vi "Read Waveform data.vi"(8 "error in (no error)":errorcluster, 11 "1D wfm (DBL) Result in":refnum<class "1D wfm (DBL) Result.lvclass">) -> (0 "error out":errorcluster, 2 "Waveform data":waveform(dbl), 3 "1D wfm (DBL) Result out":refnum<class "1D wfm (DBL) Result.lvclass">)   [LabVIEW 2015, in "1D wfm (DBL) Result.lvclass"]
uses:
  1D wfm (DBL) Result.lvclass
  1D wfm (DBL) Result.lvclass/1D wfm (DBL) Result.ctl
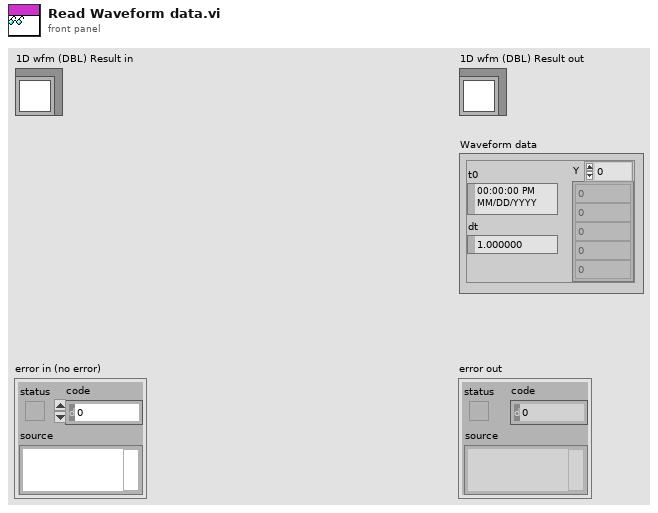
[diagram p1: front panel]
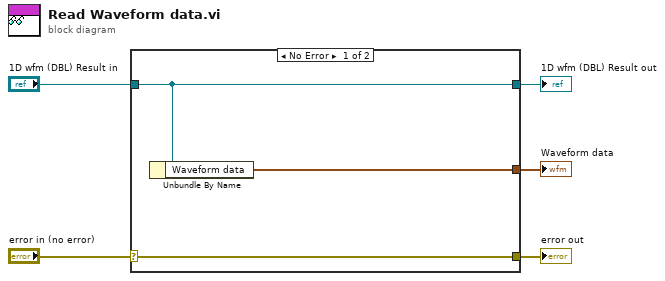
[diagram p0: block diagram]
diagram:
  n1 = case shown="No Error" "error in (no error)" {
    selector: "error in (no error)" -> [w8 w9]
    tunnel: [w8 w9] -> w4
    tunnel: [w7 w10] -> w2
    tunnel: "1D wfm (DBL) Result in" -> [w7 w10]
    tunnel: [w6 _] -> w1
    frame No Error {
      n2 = Unbundle By Name(w7) -> ("Waveform data"=w6:waveform(dbl))
    }
    frame Error {
    }
  }
  "error out" <- w4
  "1D wfm (DBL) Result out" <- w2
  "Waveform data" <- w1
